vi "Display Console.vi"(8 "error in (no error)":errorcluster) -> (0 "error out":errorcluster)   [LabVIEW 2021, in "Display Console.lvlib"]
uses:
  Display Console.lvlib
panel:
  out "PostUUT":bool
  out "PreUUT":bool
  out "Test Execution":T1
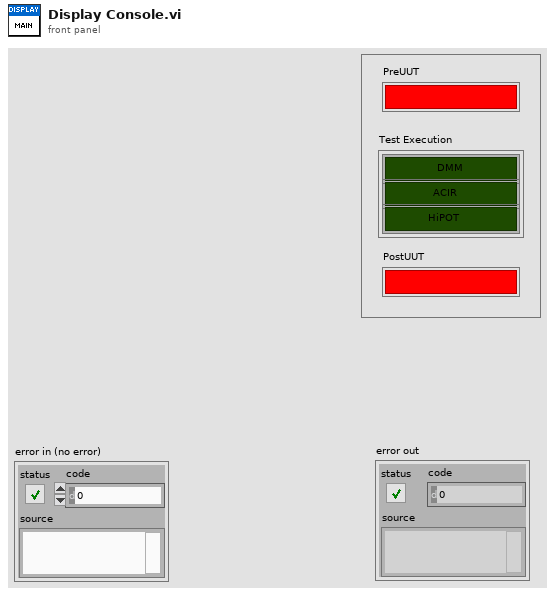
[diagram p1: front panel]
types:
  T1 = cluster{"Under body wash":bool, "bug remover":bool, "Pre-soak":bool}
  T2 = typedef "Display Console.lvlib/Module Action.ctl" = enum16{"Init", "Error", "Close"}
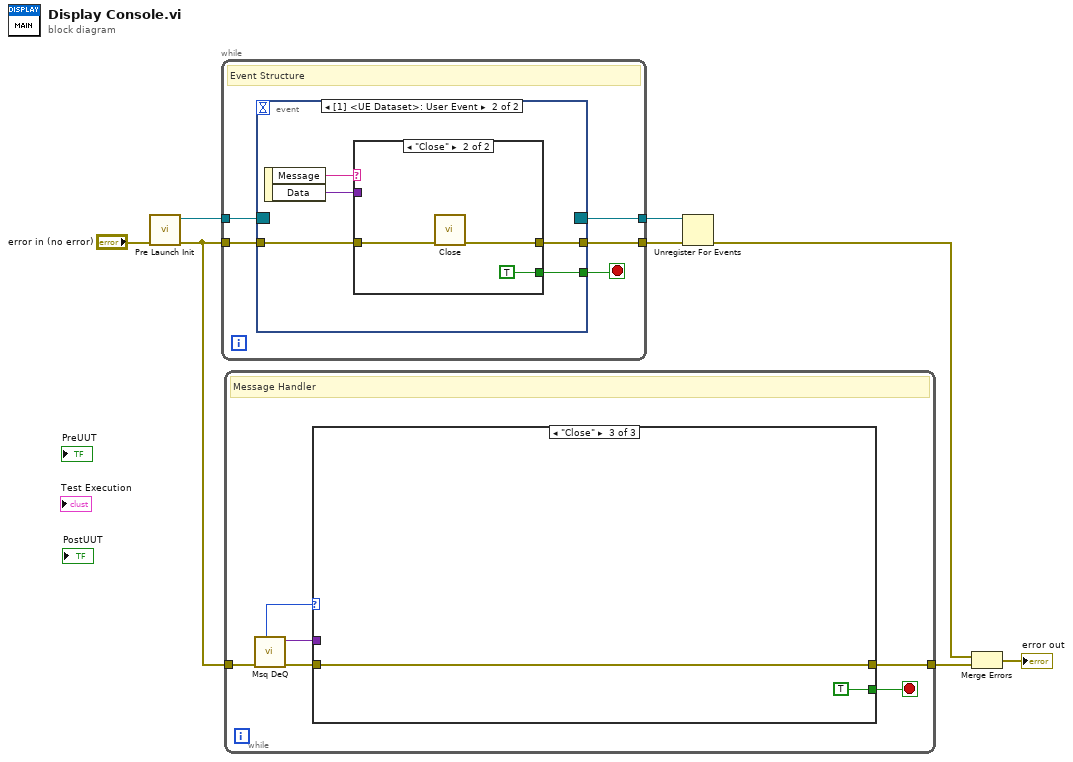
[diagram p0: block diagram]
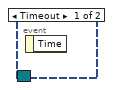
[diagram p4: hidden frame]
diagram:
  n1 = call "Pre Launch Init.vi"("error in (no error)"="error in (no error)") -> ("error out"=w2:errorcluster, "Event Registration Refnum"=w7:refnum<event-registration>)  [unwired: 9 in]
  n2 = while {
    tunnel: w2 -> [w12]
    tunnel: w7 -> [w13]
    tunnel: [w10] -> w6
    tunnel: [w9] -> w5
    stop <- w11 stop-if-true
    # "Event Structure"
    n3 = event shown="[1] <UE Dataset>: User Event" {
      selector: w13 -> [_ _]
      dyn-events: [_ _] -> w9
      timeout: _ -> [_ _]
      tunnel: w12 -> [_ w16]
      tunnel: [_ w15] -> w10
      tunnel: [_ w14] -> w11
      event Timeout {
        n4 = event-data() -> ()  [unwired: 1 in, 1 out]
      }
      event User Event {
        n5 = event-data() -> ("Message"=w18:string, "Data"=w17:variant)  [unwired: 1 in]
        n6 = case shown="\"Close\"" w18 {
          tunnel: w17 -> [_ _]
          tunnel: w16 -> [w19 w22]
          tunnel: [w19 w21] -> w15
          tunnel: [_ TRUE] -> w14
          frame Default {
          }
          frame "Close" {
            n7 = call "Close.vi"("error in (no error)"=w22) -> ("error out"=w21:errorcluster)  [unwired: 10 in]
          }
        }
      }
    }
  }
  n8 = while {
    tunnel: w2 -> [w28]
    tunnel: [w23] -> w1
    stop <- w24 stop-if-true
    # "Message Handler"
    n9 = call "Msq DeQ.vi"("error in (no error)"=w28) -> ("error out"=w26:errorcluster, "Data"=w25:variant, "Module Action"=w27:T2)  [unwired: 8 in]
    n10 = case shown="\"Close\"" w27 {
      tunnel: w26 -> [_ _ w29]
      tunnel: w25 -> [_ _ _]
      tunnel: [_ _ TRUE] -> w24
      tunnel: [_ _ w29] -> w23
      frame "Init", Default {
      }
      frame "Error" {
      }
      frame "Close" {
      }
    }
  }
  n11 = Unregister For Events(event registration refnum=w5, error in=w6) -> (error out=w4:errorcluster)
  n12 = Merge Errors(w4, w1) -> (→"error out":errorcluster)
